vi "Level Monitor.vi"(11 "App Data":T1={"Pump Station Controls"={"Lag Pump"=enum."OFF", "Lead Pump"=enum."OFF", "ALARM"=0.0, "LAG"=0.0, "LEAD"=0.0, "STOP"=0.0}, "Pump Indicators"={"Pump Water Level"=0.0, "ALARM"=FALSE, "LAG"=FALSE, "LEAD"=FALSE, "STOP"=FALSE, "PUMP 1 STATE"=FALSE, "PUMP 2 STATE"=FALSE}, "Alarm"=refnum, "Lag Start Time"=timestamp(0 s since 1904-01-01), "Lead Start Time"=timestamp(0 s since 1904-01-01), "Main Q"=refnum} {"Pump Indicators"."Pump Water Level" scale=0.0..4.0}) -> (2 "Sensor Change":bool, 3 "App Data 2":T1={"Pump Station Controls"={"Lag Pump"=enum."OFF", "Lead Pump"=enum."OFF", "ALARM"=0.0, "LAG"=0.0, "LEAD"=0.0, "STOP"=0.0}, "Pump Indicators"={"Pump Water Level"=0.0, "ALARM"=FALSE, "LAG"=FALSE, "LEAD"=FALSE, "STOP"=FALSE, "PUMP 1 STATE"=FALSE, "PUMP 2 STATE"=FALSE}, "Alarm"=refnum, "Lag Start Time"=timestamp(0 s since 1904-01-01), "Lead Start Time"=timestamp(0 s since 1904-01-01), "Main Q"=refnum} {"Pump Indicators"."Pump Water Level" scale=0.0..4.0})   [LabVIEW 2024]
uses:
  App Data.ctl
  Pump Controls.ctl
  Pump Switch.ctl
  Pump Indicators.ctl
  Q Info.ctl
  aa829e25-ffcf-4d6d-ae5f-0c87c1d4752d.vi
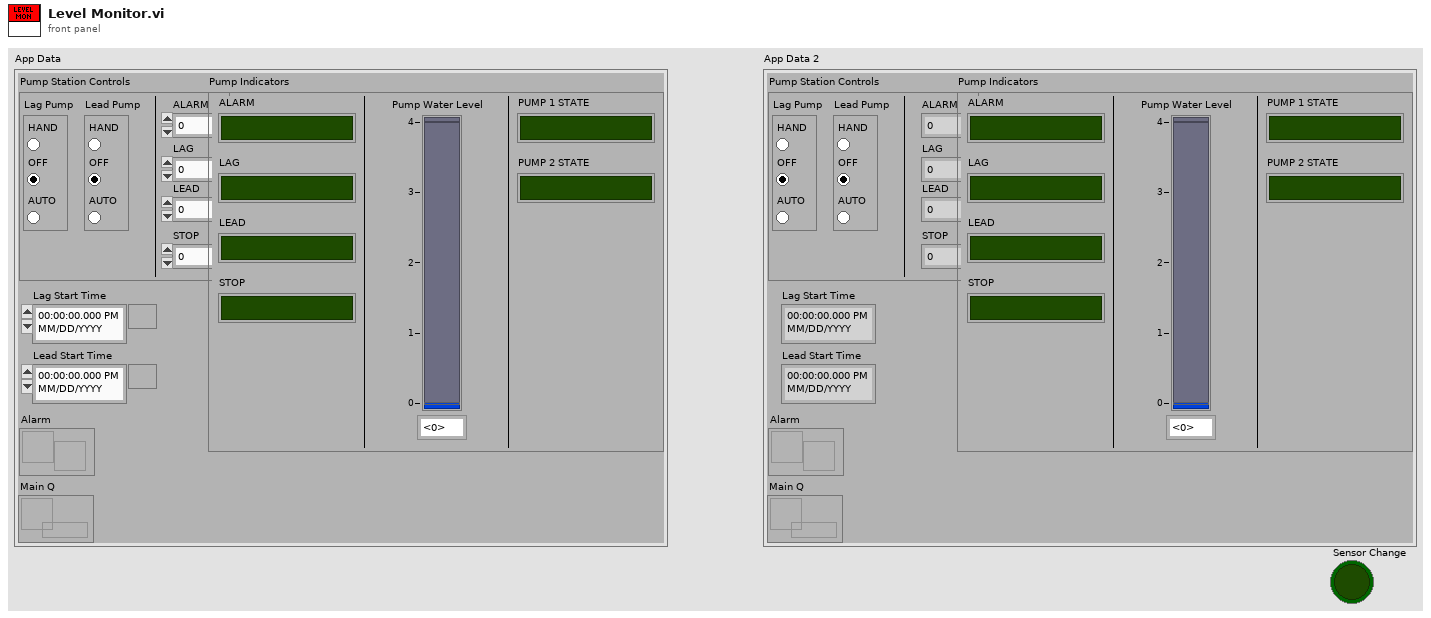
[diagram p1: front panel]
types:
  T1 = typedef "App Data.ctl" = cluster{"Pump Station Controls":T2, "Pump Indicators":T4, "Alarm":refnum<notifier>, "Lag Start Time":timestamp, "Lead Start Time":timestamp, "Main Q":refnum<queue>}
  T2 = typedef "Pump Controls.ctl" = cluster{"Lag Pump":T3, "Lead Pump":T3, "ALARM":dbl, "LAG":dbl, "LEAD":dbl, "STOP":dbl}
  T3 = typedef "Pump Switch.ctl" = enum32{"HAND", "OFF", "AUTO"}
  T4 = typedef "Pump Indicators.ctl" = cluster{"Pump Water Level":dbl, "ALARM":bool, "LAG":bool, "LEAD":bool, "STOP":bool, "PUMP 1 STATE":bool, "PUMP 2 STATE":bool}
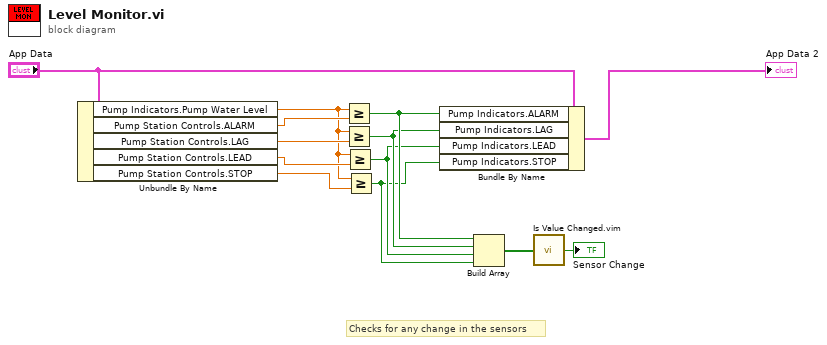
[diagram p0: block diagram]
diagram:
  # "Checks for any change in the sensors"
  n1 = Unbundle By Name("App Data") -> ("Pump Indicators.Pump Water Level"=w9:dbl, "Pump Station Controls.ALARM"=w12:dbl, "Pump Station Controls.LAG"=w11:dbl, "Pump Station Controls.LEAD"=w10:dbl, "Pump Station Controls.STOP"=w8:dbl)
  n2 = Greater Or Equal?(x=w9, y=w12) -> (x >= y?=w4:bool)
  n3 = Greater Or Equal?(x=w9, y=w11) -> (x >= y?=w3:bool)
  n4 = Greater Or Equal?(x=w9, y=w10) -> (x >= y?=w2:bool)
  n5 = Greater Or Equal?(x=w9, y=w8) -> (x >= y?=w1:bool)
  n6 = Bundle By Name(cluster="App Data", "Pump Indicators.ALARM"=w4, "Pump Indicators.LAG"=w3, "Pump Indicators.LEAD"=w2, "Pump Indicators.STOP"=w1) -> (→"App Data 2":T1)
  n7 = Build Array(w4, w3, w2, w1) -> (w7:bool[])
  n8 = call "Is Value Changed.vim"("value"=w7) -> ("changed or first call?"=→"Sensor Change":bool)
